vi "HighSpeedAverage4.vi"(0 "x 1":fxp<+/-,16,14>, 5 "x 2":fxp<+/-,16,14>, 7 "x 3":fxp<+/-,16,14>, 9 "x 4":fxp<+/-,16,14>, 11 "input valid":bool=TRUE) -> (4 "average":fxp<+/-,16,14>, 15 "output valid":bool)   [LabVIEW 2013]
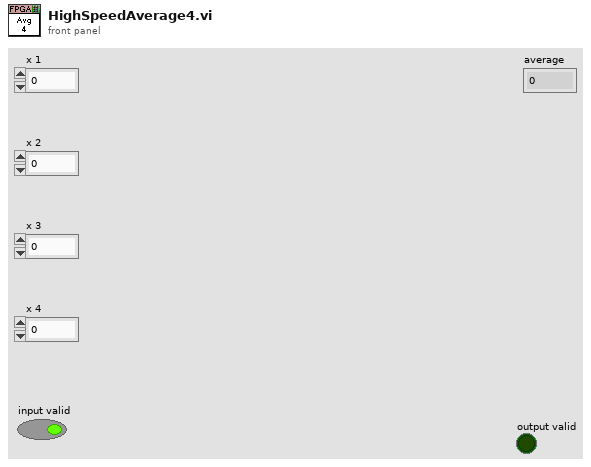
[diagram p1: front panel]
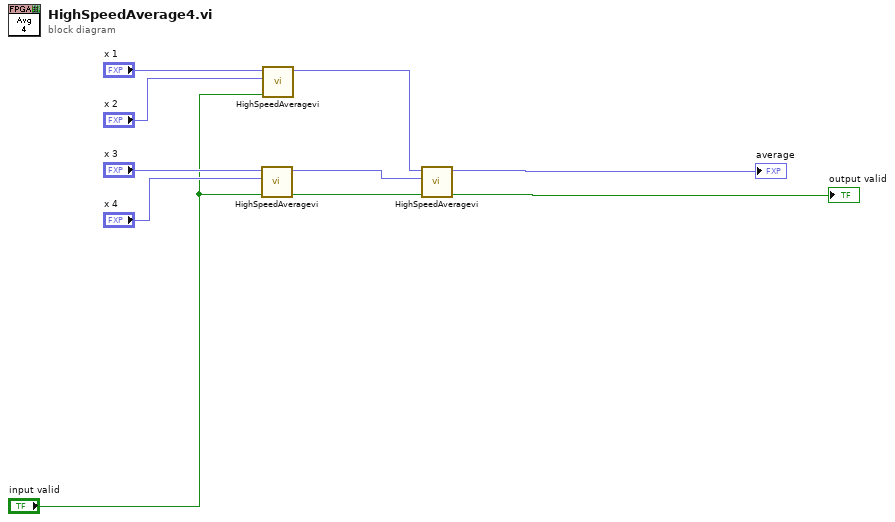
[diagram p0: block diagram]
diagram:
  n1 = call "HighSpeedAveragevi.vi"("input valid"="input valid", "y"="x 4", "x"="x 3") -> ("output valid"=w5:bool, "(x+y)/2"=w4:fxp<+/-,16,14>)  [unwired: 7 in]
  n2 = call "HighSpeedAveragevi.vi"("input valid"="input valid", "y"="x 2", "x"="x 1") -> ("(x+y)/2"=w6:fxp<+/-,16,14>)  [unwired: 7 in, 1 out]
  n3 = call "HighSpeedAveragevi.vi"("input valid"=w5, "y"=w4, "x"=w6) -> ("output valid"=→"output valid":bool, "(x+y)/2"=→"average":fxp<+/-,16,14>)  [unwired: 7 in]
